vi "FlagToRing-Keymod.vi"() -> ()   [LabVIEW 2024]
uses:
  <vilib>/regexp/Match Regular Expression.xnode
panel:
  in  "flags (0)":u16(ring) items=["SDL_KMOD_NONE"=0, "SDL_KMOD_LSHIFT"=1, "SDL_KMOD_RSHIFT"=2, "SDL_KMOD_LCTRL"=64, "SDL_KMOD_RCTRL"=128, "SDL_KMOD_LALT"=256, "SDL_KMOD_RALT"=512, "SDL_KMOD_LGUI"=1024, "SDL_KMOD_RGUI"=2048, "SDL_KMOD_NUM"=4096, "SDL_KMOD_CAPS"=8192, "SDL_KMOD_MODE"=16384, "SDL_KMOD_SCROLL"=32768, "SDL_KMOD_CTRL"=192, "SDL_KMOD_SHIFT"=3, "SDL_KMOD_ALT"=768, "SDL_KMOD_GUI"=3072]
  in  "#Define list":string="#define SDL_KMOD_NONE   0x0000u /**< no modifier is applicable. */\n#define SDL_KMOD_LSHIFT 0x0001u /**< the left Shift key is down. */\n#define SDL_KMOD_RSHIFT 0x0002u /**< the right Shift key is down. */\n#define SDL_KMOD_LCTRL  0x0040u /**< the left Ctrl (Control) key is down. */\n#define SDL_KMOD_RCTRL  0x0080u /**< the right Ctrl (Control) key is down. */\n#define SDL_KMOD_LALT   0x0100u /**< the left Alt key is down. */\n#define SDL_KMOD_RALT   0x0200u /**< the right Alt key is down. */\n#define SDL_KMOD_LGUI   0x0400u /**< the left GUI key (often the Windows key) is down. */\n#define SDL_KMOD_RGUI   0x0800u /**< the right GUI key (often the Windows key) is down. */\n#define SDL_KMOD_NUM    0x1000u /**< the Num Lock key (may be located on an extended keypad) is down. */\n#define SDL_KMOD_CAPS   0x2000u /**< the Caps Lock key is down. */\n#define SDL_KMOD_MODE   0x4000u /**< the !AltGr key is down. */\n#define SDL_KMOD_SCROLL 0x8000u /**< the Scroll Lock key is down. */\n#define SDL_KMOD_CTRL   (SDL_KMOD_LCTRL | SDL_KMOD_RCTRL)   /**< Any Ctrl key is down. */\n#define SDL_KMOD_SHIFT  (SDL_KMOD_LSHIFT | SDL_KMOD_RSHIFT) /**< Any Shift key is down. */\n#define SDL_KMOD_ALT    (SDL_KMOD_LALT | SDL_KMOD_RALT)     /**< Any Alt key is down. */\n#define SDL_KMOD_GUI    (SDL_KMOD_LGUI | SDL_KMOD_RGUI)     /**< Any GUI key is down. */"
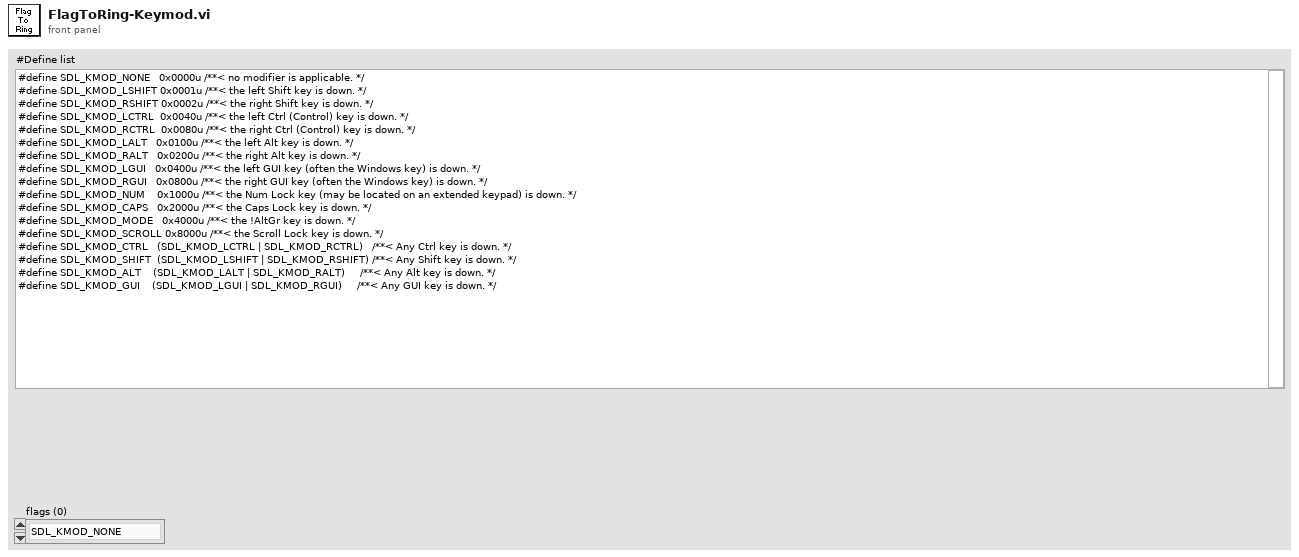
[diagram p1: front panel]
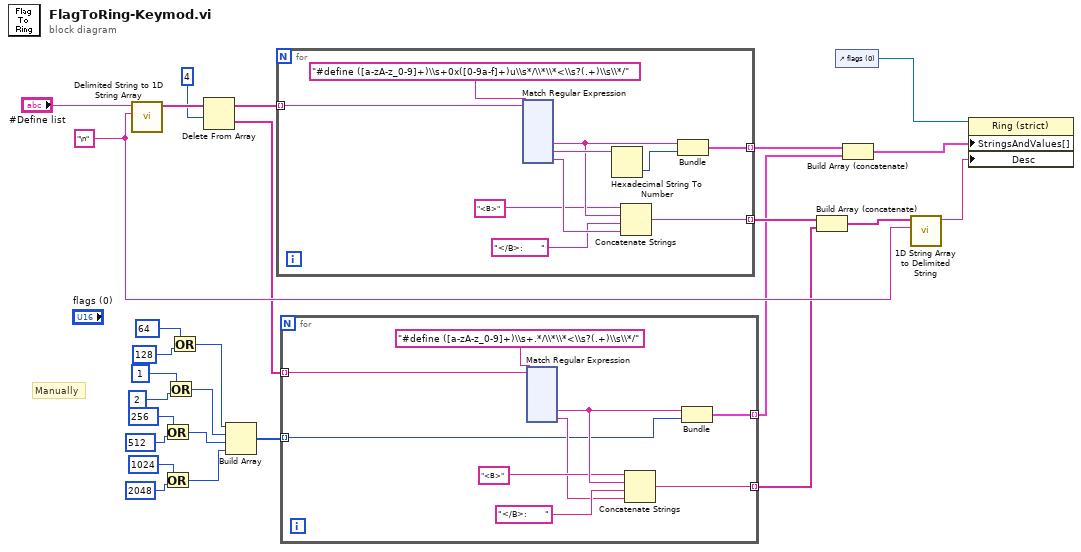
[diagram p0: block diagram]
diagram:
  w23 = "\n" ("delimiter")
  # "Manually"
  n1 = call <vilib>:"Delimited String to 1D String Array.vi"("delimiter"=w23, "delimited string"="#Define list") -> ("string array"=w26:string[])  [unwired: 9 in]
  n2 = Or(x=256 ("Numeric"), y=512 ("Numeric")) -> (x .or. y?=w5:i32)
  n3 = Or(x=1024 ("Numeric"), y=2048 ("Numeric")) -> (x .or. y?=w4:i32)
  n4 = Or(x=1 ("Numeric"), y=2 ("Numeric")) -> (x .or. y?=w6:i32)
  n5 = Or(x=64 ("Numeric"), y=128 ("Numeric")) -> (x .or. y?=w15:i32)
  n6 = Delete From Array(array=w26, length=4) -> (deleted portion=w17:string[], array with subset deleted=w19:string[])  [unwired: 1 in]
  n7 = Build Array(w15, w6, w5, w4) -> (w16:i32[])
  n8 = for {
    tunnel: w19 -> [w37] mode=indexing
    tunnel: [w34] -> w25 mode=indexing
    tunnel: [w30] -> w24 mode=indexing
    n9 = xnode "Match Regular Expression"("input string"=w37, "regular expression"="#define ([a-zA-z_0-9]+)\\s+0x([0-9a-f]+)u\\s*/\\*\\*<\\s?(.+)\\s\\*/") -> ("submatch 1"=w32:string, "submatch 2"=w35:string, "submatch 3"=w31:string)  [unwired: 4 in, 5 out]
    n10 = Hexadecimal String To Number(string=w35) -> (number=w33:u32)  [unwired: 2 in, 1 out]
    n11 = Concatenate Strings("<B>" ("string"), w32, "</B>:      " ("string"), w31) -> (w30:string)
    n12 = Bundle("submatch 1"=w32, w33) -> (w34:cluster{"submatch 1":string, u32})  [unwired: 1 in]
  }
  n13 = for {
    tunnel: w17 -> [w167] mode=indexing
    tunnel: [w165] -> w3 mode=indexing
    tunnel: [w163] -> w1 mode=indexing
    tunnel: w16 -> [w159] mode=indexing
    n14 = xnode "Match Regular Expression"("input string"=w167, "regular expression"="#define ([a-zA-z_0-9]+)\\s+.*/\\*\\*<\\s?(.+)\\s\\*/") -> ("submatch 1"=w164:string, "submatch 2"=w160:string)  [unwired: 4 in, 5 out]
    n15 = Concatenate Strings("<B>" ("string"), w164, "</B>:      " ("string"), w160) -> (w163:string)
    n16 = Bundle("submatch 1"=w164, w159) -> (w165:cluster{"submatch 1":string, i32})  [unwired: 1 in]
  }
  n17 = Build Array (concatenate)(w24, w1) -> (w2:string[])
  n18 = control-ref of="flags (0)"() -> (w22:refnum<vi>)
  n19 = Build Array (concatenate)(w25, w3) -> (w21:cluster{"submatch 1":string, u32}[])
  n20 = call <vilib>:"1D String Array to Delimited String.vi"("delimiter"=w23, "string array"=w2) -> ("delimited string"=w20:string)  [unwired: 9 in]
  n21 = property class="Ring (strict)"(reference=w22, "StringsAndValues[]"=w21, "Desc"=w20) -> ()  [unwired: 1 in, 2 out]
